vi "ReplaceOrCreateFilesSpreedSheet.vi"() -> ()   [LabVIEW 2019]
panel:
  out "error out":errorcluster
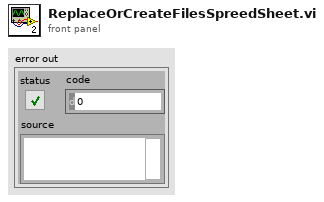
[diagram p1: front panel]
types:
  T1 = enum16{"open", "replace", "create", "open or create", "replace or create", "replace or create with confirmation"}
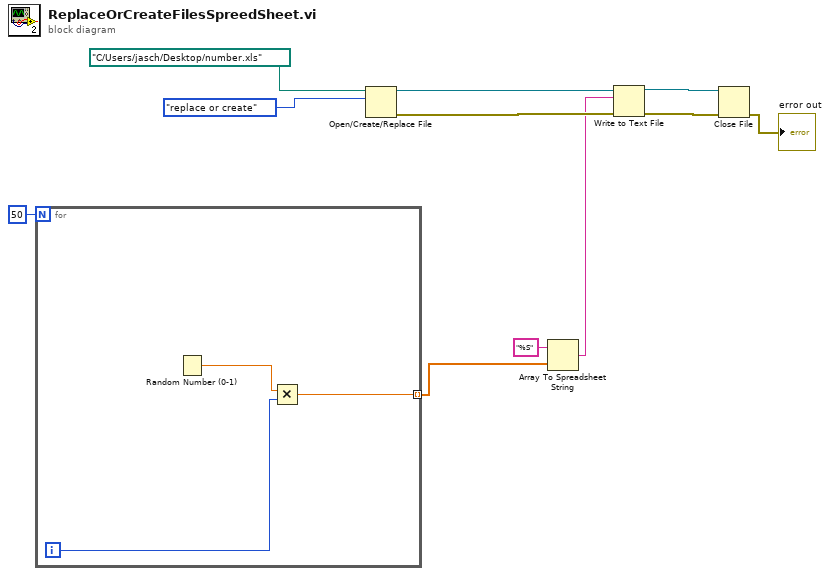
[diagram p0: block diagram]
diagram:
  n1 = for {
    N: 50 -> [_]
    tunnel: [w12] -> w10 mode=indexing
    i -> [w13]
    n2 = Random Number (0-1)() -> (number: 0 to 1=w14:dbl)
    n3 = Multiply(x=w14, y=w13) -> (x*y=w12:dbl)
  }
  n4 = Open/Create/Replace File(file path (use dialog)=path "C:/Users/jasch/Desktop/number.xls", operation (0:open)=T1."replace or create") -> (refnum out=w2:refnum<file>, error out=w6:errorcluster)  [unwired: 4 in, 1 out]
  n5 = Array To Spreadsheet String(array=w10, 3:"%S" ("format string")) -> (spreadsheet string=w5:string)  [unwired: 1 in]
  n6 = Write to Text File(file (use dialog)=w2, text=w5, error in=w6) -> (refnum out=w4:refnum<file>, error out=w3:errorcluster)  [unwired: 1 in, 1 out]
  n7 = Close File(refnum=w4, error in=w3) -> (error out=→"error out":errorcluster)  [unwired: 1 out]
